vi "Page Sixe pointsV2.vi"() -> ()   [LabVIEW 2019]
uses:
  <userlib>/Exaprom PDF/Controls/Page Controls/Page Orientation.ctl
  <userlib>/Exaprom PDF/Controls/Page Controls/Page size.ctl
panel:
  in  "Portrait":T1(array[cluster])=[{"Name"="Custom", "Width"=nan, "Height"=nan}, {"Name"="LETTER", "Width"=612.0, "Height"=792.0}, {"Name"="NOTE", "Width"=540.0, "Height"=720.0}, {"Name"="LEGAL", "Width"=612.0, "Height"=1008.0}, {"Name"="TABLOID", "Width"=792.0, "Height"=1224.0}, {"Name"="EXECUTIVE", "Width"=522.0, "Height"=756.0}, {"Name"="POSTCARD", "Width"=283.0, "Height"=416.0}, {"Name"="A0", "Width"=2384.0, "Height"=3370.0}, {"Name"="A1", "Width"=1684.0, "Height"=2384.0}, {"Name"="A2", "Width"=1191.0, "Height"=1684.0}, {"Name"="A3", "Width"=842.0, "Height"=1191.0}, {"Name"="A4", "Width"=595.0, "Height"=842.0}, {"Name"="A5", "Width"=420.0, "Height"=595.0}, {"Name"="A6", "Width"=297.0, "Height"=420.0}, {"Name"="A7", "Width"=210.0, "Height"=297.0}, {"Name"="A8", "Width"=148.0, "Height"=210.0}, {"Name"="A9", "Width"=105.0, "Height"=148.0}, {"Name"="A10", "Width"=73.0, "Height"=105.0}, {"Name"="B0", "Width"=2834.0, "Height"=4008.0}, {"Name"="B1", "Width"=2004.0, "Height"=2834.0}, {"Name"="B2", "Width"=1417.0, "Height"=2004.0}, {"Name"="B3", "Width"=1000.0, "Height"=1417.0}, {"Name"="B4", "Width"=708.0, "Height"=1000.0}, {"Name"="B5", "Width"=498.0, "Height"=708.0}, {"Name"="B6", "Width"=354.0, "Height"=498.0}, {"Name"="B7", "Width"=249.0, "Height"=354.0}, {"Name"="B8", "Width"=175.0, "Height"=249.0}, {"Name"="B9", "Width"=124.0, "Height"=175.0}, {"Name"="B10", "Width"=87.0, "Height"=124.0}, {"Name"="ARCH_E", "Width"=2592.0, "Height"=3456.0}, {"Name"="ARCH_D", "Width"=1728.0, "Height"=2592.0}, {"Name"="ARCH_C", "Width"=1296.0, "Height"=1728.0}, {"Name"="ARCH_B", "Width"=864.0, "Height"=1296.0}, {"Name"="ARCH_A", "Width"=648.0, "Height"=864.0}, {"Name"="FLSA", "Width"=612.0, "Height"=936.0}, {"Name"="FLSE", "Width"=648.0, "Height"=936.0}, {"Name"="HALFLETTER", "Width"=396.0, "Height"=612.0}, {"Name"="_11X17", "Width"=792.0, "Height"=1224.0}, {"Name"="ID_1", "Width"=242.65, "Height"=153.0}, {"Name"="ID_2", "Width"=297.0, "Height"=210.0}, {"Name"="ID_3", "Width"=354.0, "Height"=249.0}, {"Name"="LEDGER", "Width"=1224.0, "Height"=792.0}, {"Name"="CROWN_QUARTO", "Width"=535.0, "Height"=697.0}, {"Name"="LARGE_CROWN_QUARTO", "Width"=569.0, "Height"=731.0}, {"Name"="DEMY_QUARTO", "Width"=620.0, "Height"=782.0}, {"Name"="ROYAL_QUARTO", "Width"=671.0, "Height"=884.0}, {"Name"="CROWN_OCTAVO", "Width"=348.0, "Height"=527.0}, {"Name"="LARGE_CROWN_OCTAVO", "Width"=365.0, "Height"=561.0}, {"Name"="DEMY_OCTAVO", "Width"=391.0, "Height"=612.0}, {"Name"="ROYAL_OCTAVO", "Width"=442.0, "Height"=663.0}, {"Name"="SMALL_PAPERBACK", "Width"=314.0, "Height"=504.0}, {"Name"="PENGUIN_SMALL_PAPERBACK", "Width"=314.0, "Height"=513.0}, {"Name"="PENGUIN_LARGE_PAPERBACK", "Width"=365.0, "Height"=561.0}]
  out "Page Size 2":T2 items=["Custom", "LETTER", "NOTE", "LEGAL", "TABLOID", "EXECUTIVE", "POSTCARD", "A0", "A1", "A2", "A3", "A4", "A5", "A6", "A7", "A8", "A9", "A10", "B0", "B1", "B2", "B3", "B4", "B5", "B6", "B7", "B8", "B9", "B10", "ARCH_E", "ARCH_D", "ARCH_C", "ARCH_B", "ARCH_A", "FLSA", "FLSE", "HALFLETTER", "_11X17", "ID_1", "ID_2", "ID_3", "LEDGER", "CROWN_QUARTO", "LARGE_CROWN_QUARTO", "DEMY_QUARTO", "ROYAL_QUARTO", "CROWN_OCTAVO", "LARGE_CROWN_OCTAVO", "DEMY_OCTAVO", "ROYAL_OCTAVO", "SMALL_PAPERBACK", "PENGUIN_SMALL_PAPERBACK", "PENGUIN_LARGE_PAPERBACK"]
  out "Resulting page":T4
  in  "Page Size":cluster{"Width":sgl, "Height":sgl}
  in  "Orientation":T3
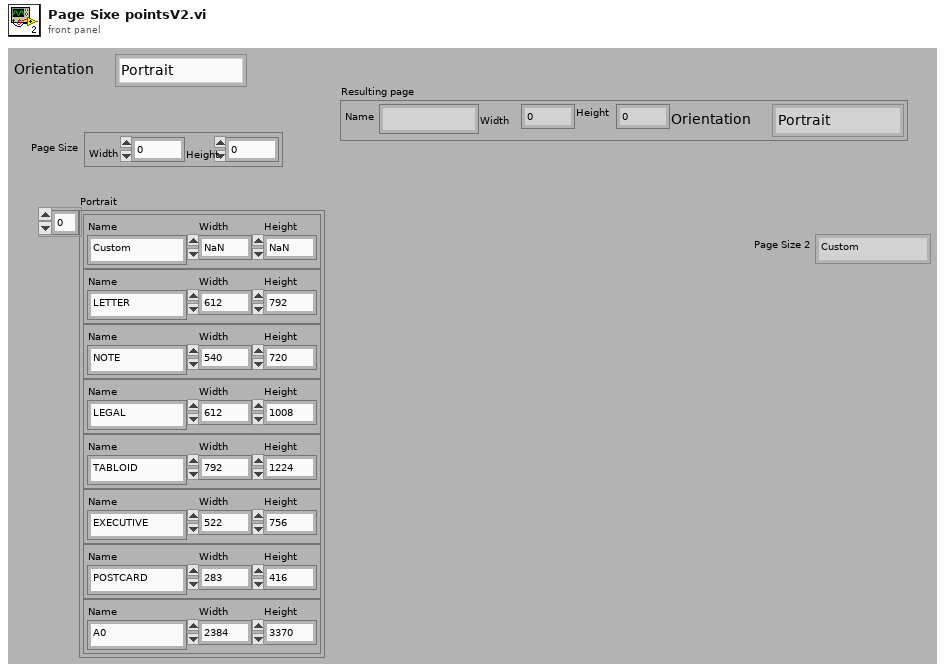
[diagram p1: front panel]
types:
  T1 = cluster{"Name":string, "Width":sgl, "Height":sgl}[]
  T2 = typedef "Page size.ctl" = i32
  T3 = typedef "Page Orientation.ctl" = enum16{"Portrait", "Landscape"}
  T4 = cluster{"Name":string, "Width":sgl, "Height":sgl, "Orientation":T3}
  T5 = cluster{"f":string, "Width":sgl, "Height":sgl, "Orientation":T3}
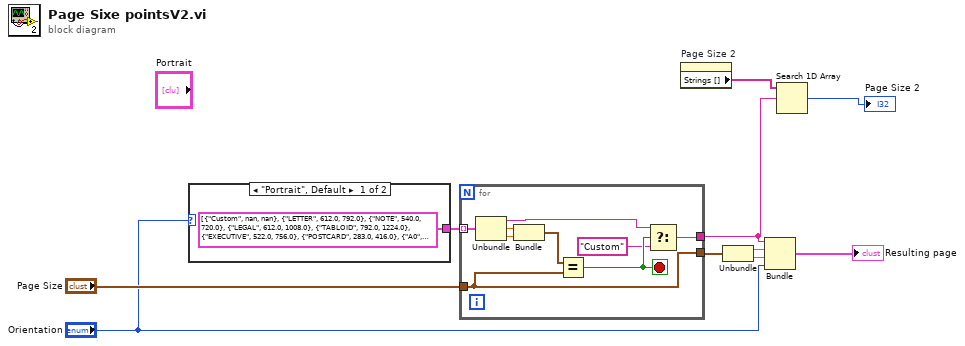
[diagram p0: block diagram]
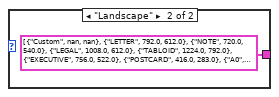
[diagram p2: hidden frame]
diagram:
  n1 = case shown="\"Portrait\", Default" "Orientation" {
    tunnel: [T1 [{"Name"="Custom", "Width"=nan, "Height"=nan}, {"Name"="LETTER", "Width"=612.0, "Height"=792.0}, {"Name"="NOTE", "Width"=540.0, "Height"=720.0}, {"Name"="LEGAL", "Width"=612.0, "Height"=1008.0}, {"Name"="TABLOID", "Width"=792.0, "Height"=1224.0}, {"Name"="EXECUTIVE", "Width"=522.0, "Height"=756.0}, {"Name"="POSTCARD", "Width"=283.0, "Height"=416.0}, {"Name"="A0", "Width"=2384.0, "Height"=3370.0}, {"Name"="A1", "Width"=1684.0, "Height"=2384.0}, {"Name"="A2", "Width"=1191.0, "Height"=1684.0}, {"Name"="A3", "Width"=842.0, "Height"=1191.0}, {"Name"="A4", "Width"=595.0, "Height"=842.0}, {"Name"="A5", "Width"=420.0, "Height"=595.0}, {"Name"="A6", "Width"=297.0, "Height"=420.0}, {"Name"="A7", "Width"=210.0, "Height"=297.0}, {"Name"="A8", "Width"=148.0, "Height"=210.0}, {"Name"="A9", "Width"=105.0, "Height"=148.0}, {"Name"="A10", "Width"=73.0, "Height"=105.0}, {"Name"="B0", "Width"=2834.0, "Height"=4008.0}, {"Name"="B1", "Width"=2004.0, "Height"=2834.0}, {"Name"="B2", "Width"=1417.0, "Height"=2004.0}, {"Name"="B3", "Width"=1000.0, "Height"=1417.0}, {"Name"="B4", "Width"=708.0, "Height"=1000.0}, {"Name"="B5", "Width"=498.0, "Height"=708.0}, {"Name"="B6", "Width"=354.0, "Height"=498.0}, {"Name"="B7", "Width"=249.0, "Height"=354.0}, {"Name"="B8", "Width"=175.0, "Height"=249.0}, {"Name"="B9", "Width"=124.0, "Height"=175.0}, {"Name"="B10", "Width"=87.0, "Height"=124.0}, {"Name"="ARCH_E", "Width"=2592.0, "Height"=3456.0}, {"Name"="ARCH_D", "Width"=1728.0, "Height"=2592.0}, {"Name"="ARCH_C", "Width"=1296.0, "Height"=1728.0}, {"Name"="ARCH_B", "Width"=864.0, "Height"=1296.0}, {"Name"="ARCH_A", "Width"=648.0, "Height"=864.0}, {"Name"="FLSA", "Width"=612.0, "Height"=936.0}, {"Name"="FLSE", "Width"=648.0, "Height"=936.0}, {"Name"="HALFLETTER", "Width"=396.0, "Height"=612.0}, {"Name"="_11X17", "Width"=792.0, "Height"=1224.0}, {"Name"="ID_1", "Width"=242.65, "Height"=153.0}, {"Name"="ID_2", "Width"=297.0, "Height"=210.0}, {"Name"="ID_3", "Width"=354.0, "Height"=249.0}, {"Name"="LEDGER", "Width"=1224.0, "Height"=792.0}, {"Name"="CROWN_QUARTO", "Width"=535.0, "Height"=697.0}, {"Name"="LARGE_CROWN_QUARTO", "Width"=569.0, "Height"=731.0}, {"Name"="DEMY_QUARTO", "Width"=620.0, "Height"=782.0}, {"Name"="ROYAL_QUARTO", "Width"=671.0, "Height"=884.0}, {"Name"="CROWN_OCTAVO", "Width"=348.0, "Height"=527.0}, {"Name"="LARGE_CROWN_OCTAVO", "Width"=365.0, "Height"=561.0}, {"Name"="DEMY_OCTAVO", "Width"=391.0, "Height"=612.0}, {"Name"="ROYAL_OCTAVO", "Width"=442.0, "Height"=663.0}, {"Name"="SMALL_PAPERBACK", "Width"=314.0, "Height"=504.0}, {"Name"="PENGUIN_SMALL_PAPERBACK", "Width"=314.0, "Height"=513.0}, {"Name"="PENGUIN_LARGE_PAPERBACK", "Width"=365.0, "Height"=561.0}] ("Portrait") T1 [{"Name"="Custom", "Width"=nan, "Height"=nan}, {"Name"="LETTER", "Width"=792.0, "Height"=612.0}, {"Name"="NOTE", "Width"=720.0, "Height"=540.0}, {"Name"="LEGAL", "Width"=1008.0, "Height"=612.0}, {"Name"="TABLOID", "Width"=1224.0, "Height"=792.0}, {"Name"="EXECUTIVE", "Width"=756.0, "Height"=522.0}, {"Name"="POSTCARD", "Width"=416.0, "Height"=283.0}, {"Name"="A0", "Width"=3370.0, "Height"=2384.0}, {"Name"="A1", "Width"=2384.0, "Height"=1684.0}, {"Name"="A2", "Width"=1684.0, "Height"=1191.0}, {"Name"="A3", "Width"=1191.0, "Height"=842.0}, {"Name"="A4", "Width"=842.0, "Height"=595.0}, {"Name"="A5", "Width"=595.0, "Height"=420.0}, {"Name"="A6", "Width"=420.0, "Height"=297.0}, {"Name"="A7", "Width"=297.0, "Height"=210.0}, {"Name"="A8", "Width"=210.0, "Height"=148.0}, {"Name"="A9", "Width"=148.0, "Height"=105.0}, {"Name"="A10", "Width"=105.0, "Height"=73.0}, {"Name"="B0", "Width"=4008.0, "Height"=2834.0}, {"Name"="B1", "Width"=2834.0, "Height"=2004.0}, {"Name"="B2", "Width"=2004.0, "Height"=1417.0}, {"Name"="B3", "Width"=1417.0, "Height"=1000.0}, {"Name"="B4", "Width"=1000.0, "Height"=708.0}, {"Name"="B5", "Width"=708.0, "Height"=498.0}, {"Name"="B6", "Width"=498.0, "Height"=354.0}, {"Name"="B7", "Width"=354.0, "Height"=249.0}, {"Name"="B8", "Width"=249.0, "Height"=175.0}, {"Name"="B9", "Width"=175.0, "Height"=124.0}, {"Name"="B10", "Width"=124.0, "Height"=87.0}, {"Name"="ARCH_E", "Width"=3456.0, "Height"=2592.0}, {"Name"="ARCH_D", "Width"=2592.0, "Height"=1728.0}, {"Name"="ARCH_C", "Width"=1728.0, "Height"=1296.0}, {"Name"="ARCH_B", "Width"=1296.0, "Height"=864.0}, {"Name"="ARCH_A", "Width"=864.0, "Height"=648.0}, {"Name"="FLSA", "Width"=936.0, "Height"=612.0}, {"Name"="FLSE", "Width"=936.0, "Height"=648.0}, {"Name"="HALFLETTER", "Width"=612.0, "Height"=396.0}, {"Name"="_11X17", "Width"=1224.0, "Height"=792.0}, {"Name"="ID_1", "Width"=153.0, "Height"=242.65}, {"Name"="ID_2", "Width"=210.0, "Height"=297.0}, {"Name"="ID_3", "Width"=249.0, "Height"=354.0}, {"Name"="LEDGER", "Width"=792.0, "Height"=1224.0}, {"Name"="CROWN_QUARTO", "Width"=697.0, "Height"=535.0}, {"Name"="LARGE_CROWN_QUARTO", "Width"=731.0, "Height"=569.0}, {"Name"="DEMY_QUARTO", "Width"=782.0, "Height"=620.0}, {"Name"="ROYAL_QUARTO", "Width"=884.0, "Height"=671.0}, {"Name"="CROWN_OCTAVO", "Width"=527.0, "Height"=348.0}, {"Name"="LARGE_CROWN_OCTAVO", "Width"=561.0, "Height"=365.0}, {"Name"="DEMY_OCTAVO", "Width"=612.0, "Height"=391.0}, {"Name"="ROYAL_OCTAVO", "Width"=663.0, "Height"=442.0}, {"Name"="SMALL_PAPERBACK", "Width"=504.0, "Height"=314.0}, {"Name"="PENGUIN_SMALL_PAPERBACK", "Width"=513.0, "Height"=314.0}, {"Name"="PENGUIN_LARGE_PAPERBACK", "Width"=561.0, "Height"=365.0}] ("Landscape")] -> w10
    frame "Portrait", Default {
    }
    frame "Landscape" {
    }
  }
  n2 = for {
    tunnel: w10 -> [w21] mode=indexing
    tunnel: "Page Size" -> [w13]
    tunnel: [w14] -> w2
    tunnel: [w13] -> w8
    stop <- w17 stop-if-true
    n3 = Unbundle(w21) -> ("Name"=w15:string, "Width"=w20:sgl, "Height"=w19:sgl)
    n4 = Bundle("Width"=w20, "Height"=w19) -> (w18:cluster{"Width":sgl, "Height":sgl})  [unwired: 1 in]
    n5 = Equal?(x=w18, y=w13) -> (x = y?=w17:bool)
    n6 = Select(t=w15, s=w17, f="Custom") -> (s? t:f=w14:string)
  }
  n7 = property on="Page Size 2" class="Ring (strict)"() -> ("Strings []"=w3:string[])  [unwired: 2 in, 2 out]
  n8 = Unbundle(w8) -> ("Width"=w7:sgl, "Height"=w6:sgl)
  n9 = Bundle("f"=w2, "Width"=w7, "Height"=w6, "Orientation"="Orientation") -> (→"Resulting page":T5)  [unwired: 1 in]
  n10 = Search 1D Array(1D array=w3, element=w2) -> (index of element=→"Page Size 2":i32)  [unwired: 1 in]
